vi "Process Name.vi"() -> (3 "process name":string)   [LabVIEW 2021, in "AnalogGeneration.lvlib"]
uses:
  AnalogGeneration.lvlib
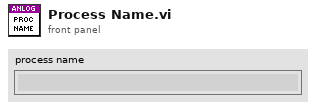
[diagram p1: front panel]
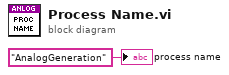
[diagram p0: block diagram]
diagram:
  "process name" <- "AnalogGeneration" ("ProcessName")
